vi "Read Succeed State .vi"(8 "error in (no error)":errorcluster, 11 "Test Boolean in":refnum<class "Test Boolean.lvclass">) -> (0 "error out":errorcluster, 2 "Succeed State":T1, 3 "Test Boolean out":refnum<class "Test Boolean.lvclass">)   [LabVIEW 2021, in "BT.lvlib" / "Test Boolean.lvclass"]
uses:
  Test Boolean.lvclass
  abs_Test Boolean/Support/Succeed State.ctl
  Test Boolean.lvclass/Test Boolean.ctl
  abs_Test Boolean/abs_Test Boolean.lvclass
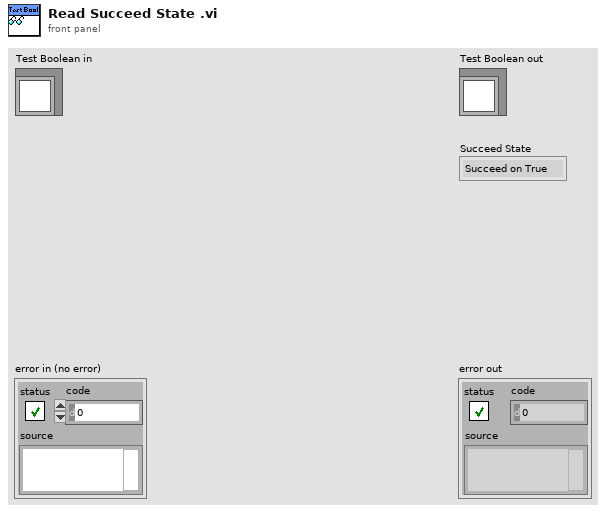
[diagram p1: front panel]
types:
  T1 = typedef "BT.lvlib/abs_Test Boolean.lvclass/Succeed State.ctl" = enum16{"Succeed on True", "Succeed on Fail"}
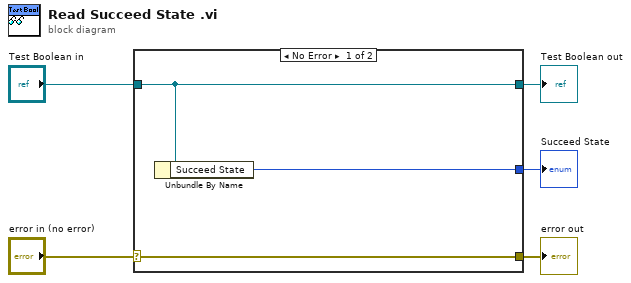
[diagram p0: block diagram]
diagram:
  n1 = case shown="No Error" "error in (no error)" {
    selector: "error in (no error)" -> [w8 w9]
    tunnel: [w8 w9] -> w4
    tunnel: [w7 w10] -> w2
    tunnel: "Test Boolean in" -> [w7 w10]
    tunnel: [w6 _] -> w1
    frame No Error {
      n2 = Unbundle By Name(w7) -> ("Succeed State"=w6:T1)
    }
    frame Error {
    }
  }
  "error out" <- w4
  "Test Boolean out" <- w2
  "Succeed State" <- w1
